vi "Runner.FilterRunnerCallers.vi"(10 "Paths":path[](array[path])) -> (2 "Filtered Paths":path[](array[path]))   [LabVIEW 2013, in "Caraya.lvlib" / "Test Runner.lvclass"]
uses:
  Test Runner.lvclass
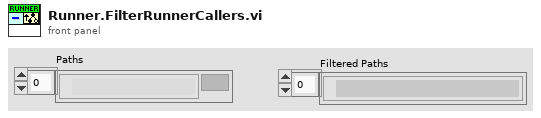
[diagram p1: front panel]
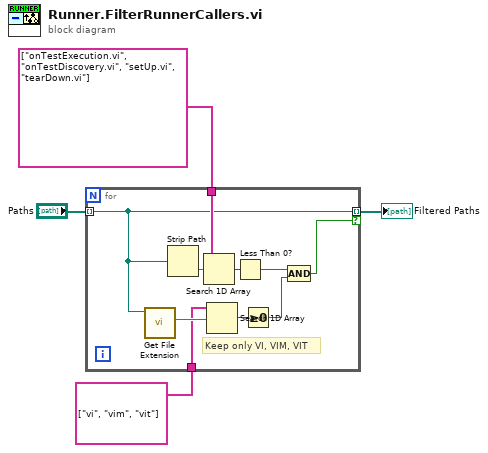
[diagram p0: block diagram]
diagram:
  n1 = for {
    tunnel: [w5] -> w2 mode=indexing if=w13
    tunnel: string[] ["vi", "vim", "vit"] -> [w11]
    tunnel: string[] ["onTestExecution.vi", "onTestDiscovery.vi", "setUp.vi", "tearDown.vi"] -> [w9]
    tunnel: "Paths" -> [w5] mode=indexing
    # "Keep only VI, VIM, VIT"
    n2 = call <vilib>:"Get File Extension.vi"("file"=w5) -> ("lowercase file extension"=w12:string)  [unwired: 7 in, 3 out]
    n3 = Strip Path(path=w5) -> (name=w8:string)  [unwired: 1 out]
    n4 = Search 1D Array(1D array=w9, element=w8) -> (index of element=w7:i32)  [unwired: 1 in]
    n5 = Search 1D Array(1D array=w11, element=w12) -> (index of element=w14:i32)  [unwired: 1 in]
    n6 = Less Than 0?(x=w7) -> (x < 0?=w6:bool)
    n7 = Greater Or Equal To 0?(x=w14) -> (x >= 0?=w10:bool)
    n8 = Compound Arithmetic op=AND(w6, w10) -> (w13:bool)
  }
  "Filtered Paths" <- w2
